vi "Trajectory Adaptation Algorithm_v2.vi"(0 "start (xi,yi)":dbl[](array[numeric])=[0.0, 5.0] format="%.2f", 1 "baseline (x,y)":dbl[](array[numeric])=[0.0, 5.0] format="%.2f", 5 "(r_eye,r_assign)":dbl[](array[numeric])=[5.0, 1.0], 7 "Tassign":dbl[](array[numeric])=[0.0, 5.0], 9 "Tt":dbl, 11 "Th":dbl, 12 "index":i32) -> (4 "adapted (x,y)":dbl[](array[numeric]))   [LabVIEW 2010]
doc: "This VI transforms the current (x,y) into a new location based on the assigned radius R assign and assigned translation vector Tassign. The location is index/time dependent: the frist Tt seconds, rotation matrix and translation vector ramp up linearly, and then it would stay for another Th seconds, after that they ramp down to what they originally were and stay there unless otherwise told to.\n\nInterrupt is possible because of the additional registers added, namely, the new adaptation can be demanded while the previos one hasn't finished yet."
uses:
  <vilib>/Analysis/NI_AALBase.lvlib
  <vilib>/Analysis/baseanly.llb/A x Vector.vi
  <vilib>/Analysis/Matrix/NI_Matrix.lvlib
  <vilib>/Analysis/Matrix/Numeric/Conversions/Array To Matrix - RA2.vi
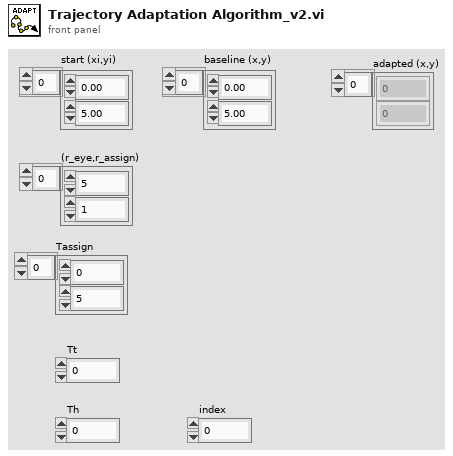
[diagram p1: front panel]
types:
  T1 = typedef "NI_Matrix.lvlib/RealMatrix.ctl" = dbl[][]
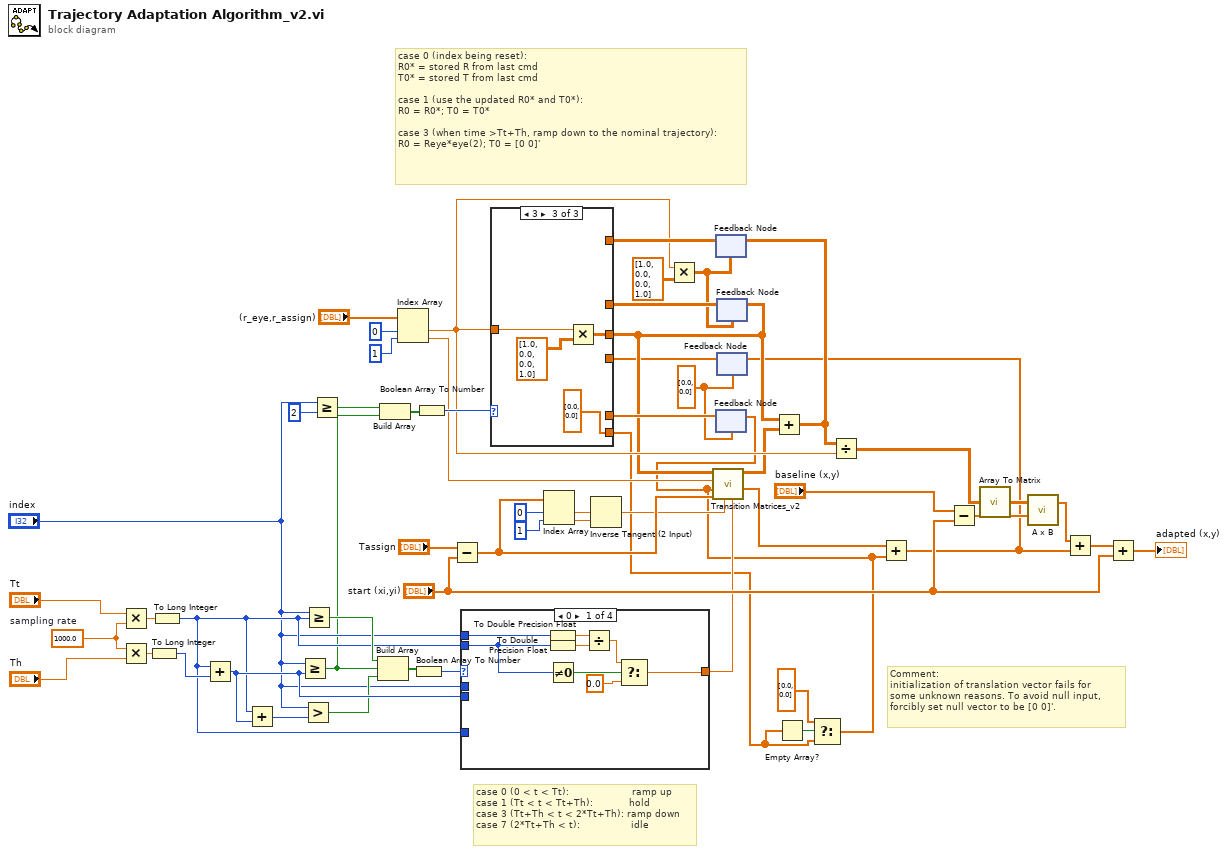
[diagram p0: block diagram]
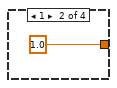
[diagram p4: hidden frame]
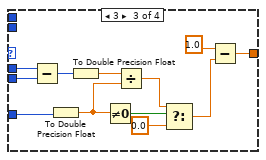
[diagram p5: hidden frame]
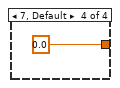
[diagram p6: hidden frame]
diagram:
  w3 = dbl[] [0.0, 0.0] ("Assign Point")
  w53 = 1000.0  # sampling rate
  # "Comment:\ninitialization of translation vector fails for\nsome unknown reasons. To avoid null input,\nforcibly set null vector to be [0 0]'."
  # "case 0 (index being reset):\nR0* = stored R from last cmd\nT0* = stored T from last cmd\n\ncase 1 (use the updated R0* and T0*):\nR0 = R0*; T0 = T0*\n\ncase 3 (when time >Tt+Th, ramp down to the nominal trajectory):\nR0 = Reye*eye(2); T0 = [0 0]'"
  # "case 0 (0 < t < Tt):                     ramp up\ncase 1 (Tt < t < Tt+Th):            hold\ncase 3 (Tt+Th < t < 2*Tt+Th): ramp down\ncase 7 (2*Tt+Th < t):                 idle"
  n1 = Multiply(x="Tt", y=w53) -> (x*y=w55:dbl)
  n2 = Multiply(x=w53, y="Th") -> (x*y=w56:dbl)
  n3 = To Long Integer(number=w56) -> (32bit integer=w54:i32)
  n4 = To Long Integer(number=w55) -> (32bit integer=w32:i32)
  n5 = Add(x=w32, y=w54) -> (x+y=w33:i32)
  n6 = Add(x=w32, y=w33) -> (x+y=w49:i32)
  n7 = Greater Or Equal?(x="index", y=w33) -> (x >= y?=w13:bool)
  n8 = Greater?(x="index", y=w49) -> (0:w30:bool)
  n9 = Greater Or Equal?(x="index", y=w32) -> (x >= y?=w52:bool)
  n10 = Greater Or Equal?(x="index", y=2) -> (x >= y?=w17:bool)
  n11 = Build Array(w52, w13, w30) -> (w51:bool[])
  n12 = Build Array(w17, w13) -> (w29:bool[])
  n13 = Index Array(array="(r_eye,r_assign)", index #1=0 ("index"), index #2=1 ("index")) -> (element #1=w19:dbl, element #2=w25:dbl)
  n14 = Boolean Array To Number(Boolean array=w51) -> (number=w50:u32)
  n15 = Boolean Array To Number(Boolean array=w29) -> (number=w28:u32)
  n16 = Subtract(x="Tassign", y="start (xi,yi)") -> (x-y=w37:dbl[])
  n17 = case shown="0" w50 {
    tunnel: w32 -> [w61 _ _ _]
    tunnel: "index" -> [w62 _ _ _]
    tunnel: [w58 1.0 w74 0.0] -> w24
    tunnel: "index" -> [_ _ w76 _]
    tunnel: w33 -> [_ _ w75 _]
    tunnel: w32 -> [_ _ w71 _]
    frame 0 {
      n18 = To Double Precision Float(number=w62) -> (double precision float=w64:dbl)
      n19 = To Double Precision Float(number=w61) -> (double precision float=w63:dbl)
      n20 = Not Equal To 0?(x=w61) -> (x != 0?=w60:bool)
      n21 = Divide(x=w64, y=w63) -> (x/y=w59:dbl)
      n22 = Select(t=w59, s=w60, f=0.0) -> (s? t:f=w58:dbl)
    }
    frame 1 {
    }
    frame 3 {
      n23 = Subtract(x=w76, y=w75) -> (x-y=w73:i32)
      n24 = To Double Precision Float(number=w71) -> (double precision float=w68:dbl)
      n25 = To Double Precision Float(number=w73) -> (double precision float=w72:dbl)
      n26 = Not Equal To 0?(x=w68) -> (x != 0?=w70:bool)
      n27 = Divide(x=w72, y=w68) -> (x/y=w66:dbl)
      n28 = Select(t=w66, s=w70, f=0.0) -> (s? t:f=w67:dbl)
      n29 = Subtract(x=1.0, y=w67) -> (x-y=w74:dbl)
    }
    frame 7, Default {
    }
  }
  n30 = Index Array(array=w37, index #1=0 ("index"), index #2=1 ("index")) -> (element #1=w45:dbl, element #2=w44:dbl)
  n31 = Inverse Tangent (2 Input)(1:w44, 2:w45) -> (0:w22:dbl)
  n32 = Multiply(x=w19, y=dbl[][] [[1.0, 0.0], [0.0, 1.0]]) -> (x*y=w15:dbl[][])
  n33 = feedback #1(w15) -> (w23:dbl[][])
  n34 = feedback #2(w3) -> (w14:dbl[])
  n35 = feedback #3(w15) -> (w16:dbl[][])
  n36 = feedback #4(w3) -> (w6:dbl[])
  n37 = case shown="3" w28 {
    tunnel: w19 -> [_ _ w85]
    tunnel: [w80 w82 w84] -> w10
    tunnel: w23 -> [w80 _ _]
    tunnel: w6 -> [w79 _ _]
    tunnel: [w79 w81 dbl[] [0.0, 0.0]] -> w2
    tunnel: w16 -> [_ w82 _]
    tunnel: w14 -> [_ w81 _]
    frame 0, Default {
    }
    frame 1 {
    }
    frame 3 {
      n38 = Multiply(x=w85, y=dbl[][] [[1.0, 0.0], [0.0, 1.0]]) -> (x*y=w84:dbl[][])
    }
  }
  n39 = feedback-in #3(w10) -> ()
  n40 = Empty Array?(array=w2) -> (empty?=w5:bool)
  n41 = Select(t=dbl[] [0.0, 0.0], s=w5, f=w2) -> (s? t:f=w1:dbl[])
  n42 = call "Transition Matrices_v2.vi"("alpha"=w24, "theta"=w22, "Tassign"=w37, "T0"=w1, "Rassign"=w25, "R0"=w10) -> ("Translation Vector"=w8:dbl[], "Rotation Matrix"=w9:dbl[][])  [unwired: 4 in]
  n43 = feedback-in #2(w1) -> ()
  n44 = Add(x=w10, y=w9) -> (x+y=w18:dbl[][])
  n45 = feedback-in #1(w18) -> ()
  n46 = Divide(x=w18, y=w19) -> (x/y=w27:dbl[][])
  n47 = Add(x=w8, y=w1) -> (x+y=w7:dbl[])
  n48 = feedback-in #4(w7) -> ()
  n49 = Subtract(x="baseline (x,y)", y="start (xi,yi)") -> (x-y=w41:dbl[])
  n50 = call-poly <vilib>:"Array To Matrix.vi"("Real 2D Array"=w27) -> ("Real Matrix"=w43:T1)
  n51 = call-poly <vilib>:"A x B.vi"("Vector"=w41, "A"=w43) -> ("A x Vector"=w48:dbl[])  [unwired: 1 out]
  n52 = Add(x=w48, y=w7) -> (x+y=w40:dbl[])
  n53 = Add(x=w40, y="start (xi,yi)") -> (x+y=→"adapted (x,y)":dbl[])
